vi "Punkte_mit_linie_verbinden.vi"(6 "Color":u32, 9 "Array":dbl[][](array[numeric]), 10 "dimension size":i32, 11 "Refnum in":T1) -> (3 "Refnum out":T1)   [LabVIEW 2014]
uses:
  <vilib>/vision/Image Controls.llb/IMAQ Image.ctl
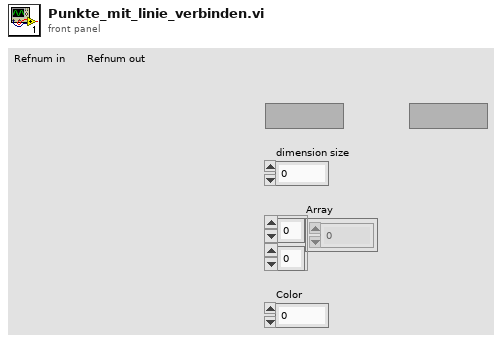
[diagram p1: front panel]
types:
  T1 = typedef "IMAQ Image.ctl" = refnum<image>
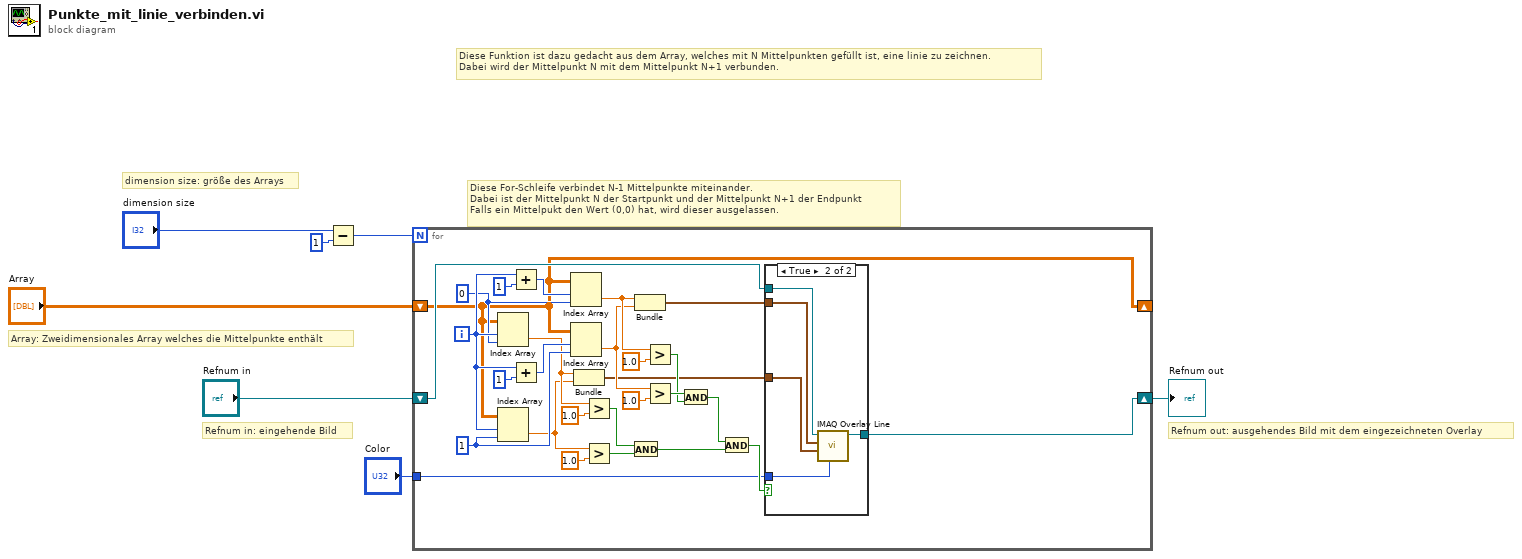
[diagram p0: block diagram]
diagram:
  # "Diese For-Schleife verbindet N-1 Mittelpunkte miteinander. \nDabei ist der Mittelpunkt N der Startpunkt und der Mittelpunkt N+1 der Endpunkt\nFalls ein Mittelpukt den Wert (0,0) hat, wird dieser ausgelassen."
  # "Refnum out: ausgehendes Bild mit dem eingezeichneten Overlay"
  # "Refnum in: eingehende Bild"
  # "Array: Zweidimensionales Array welches die Mittelpunkte enthält"
  # "dimension size: größe des Arrays"
  # "Diese Funktion ist dazu gedacht aus dem Array, welches mit N Mittelpunkten gefüllt ist, eine linie zu zeichnen. \nDabei wird der Mittelpunkt N mit dem Mittelpunkt N+1 verbunden."
  n1 = Subtract(x="dimension size", y=1) -> (x-y=w4:i32)
  n2 = for {
    N: w4 -> [_]
    shift-right: [w10] -> _
    shift-left: "Array" -> [w10]
    shift-right: [w35] -> w2
    shift-left: "Refnum in" -> [w34]
    tunnel: "Color" -> [w11]
    i -> [w33]
    w29 = 0 ("index (col)")
    w30 = 1 ("disabled index (col)")
    n3 = Index Array(array=w10, index (row)=w33, index (col)=w29) -> (element=w16:dbl)
    n4 = Index Array(array=w10, index (row)=w33, index (col)=w30) -> (element=w15:dbl)
    n5 = Add(x=w33, y=1) -> (x+y=w32:i32)
    n6 = Add(x=w33, y=1) -> (x+y=w31:i32)
    n7 = Index Array(array=w10, index (row)=w32, index (col)=w29) -> (element=w22:dbl)
    n8 = Index Array(array=w10, index (row)=w31, index (col)=w30) -> (element=w21:dbl)
    n9 = Bundle("element"=w16, "element"=w15) -> (w8:cluster{"element":dbl, "element":dbl})  [unwired: 1 in]
    n10 = Greater?(x=w16, y=1.0) -> (0:w18:bool)
    n11 = Greater?(x=w15, y=1.0) -> (0:w17:bool)
    n12 = And(x=w18, y=w17) -> (x .and. y?=w13:bool)
    n13 = Bundle("element"=w22, "element"=w21) -> (w9:cluster{"element":dbl, "element":dbl})  [unwired: 1 in]
    n14 = Greater?(x=w22, y=1.0) -> (0:w23:bool)
    n15 = Greater?(x=w21, y=1.0) -> (0:w24:bool)
    n16 = And(x=w24, y=w23) -> (x .and. y?=w14:bool)
    n17 = And(x=w14, y=w13) -> (x .and. y?=w12:bool)
    n18 = case shown="True" w12 {
      tunnel: [w36 w41] -> w35
      tunnel: w34 -> [w36 w40]
      tunnel: w8 -> [_ w37]
      tunnel: w9 -> [_ w38]
      tunnel: w11 -> [_ w39]
      frame False {
      }
      frame True {
        n19 = call "IMAQ Overlay Line"("Color"=w39, "End Point"=w37, "Start Point"=w38, "Image"=w40) -> ("Image Out"=w41:T1)  [unwired: 6 in, 1 out]
      }
    }
  }
  "Refnum out" <- w2
